vi "Load_Firmware.vi"(3 "Task":enum16{"Get Version", "Replace"}(ring), 5 "Bot Settings":T1) -> (0 "error out":errorcluster, 1 "Version":dbl, 2 "standard error":string)   [LabVIEW 2012]
uses:
  <userlib>/BotSpeak/VIs/Direct/BotSpeak_Control.ctl
panel:
  out "password":string
  out "return code":i32
  out "address":string="192.168.7.2"
  out "username":string="root"
  out "filenames":string[](array[string])=["BotSpeak2.js", "BotSpeak3.js", "BotSpeak4.js"]
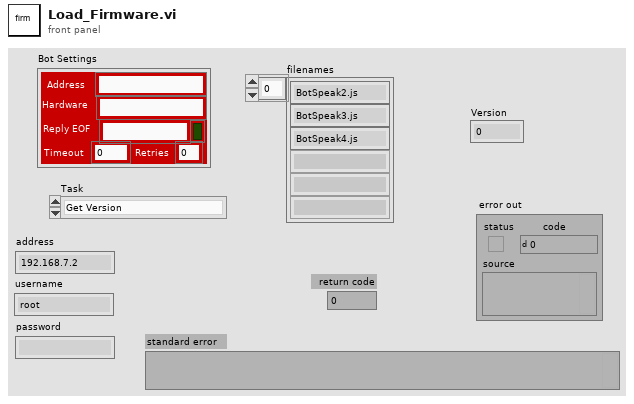
[diagram p1: front panel]
types:
  T1 = typedef "BotSpeak_Control.ctl" = cluster{"Address":string, "Reply EOF":string, "Hardware":string, "Retries":i8, "Timeout":i32, "Open?":bool}
  T2 = typedef "BotSpeak.HardwareSpecs.ctl" = cluster{"Hardware Name":string, "Hardware URL":string, "ComType":enum16{"Undefined", "Serial", "TCPIP", "Console", "EV3"}, "TCP Port":i32, "DefaultAddress":string, "Retries":i32, "Translate":enum16{"None", "Tiny", "URAPI"}, "MaxScriptSize":i32, "MaxVarNumber":i32, "StartupWait":i32, "Patience":i32, "Startup Patience":i32, "Hardware Help":string, "Com Protocol":string, "Translator":cluster{"BotSpeak CMD":string, "CMD out":string}[], "Init Code":string, "Variable Format":enum16{"INT", "FLOAT", "FIXED"}, "username":string, "password":string}
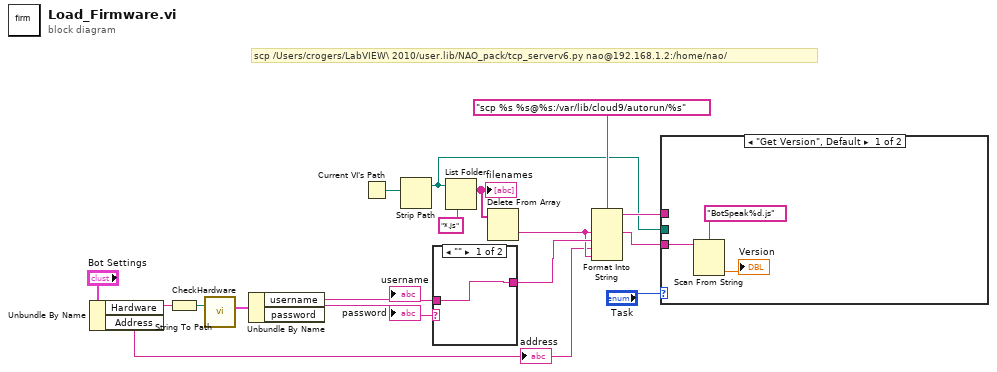
[diagram p0: block diagram]
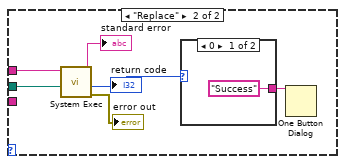
[diagram p2: hidden frame]
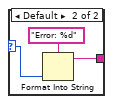
[diagram p3: hidden frame]
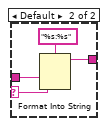
[diagram p4: hidden frame]
diagram:
  # "scp /Users/crogers/LabVIEW\\ 2010/user.lib/NAO_pack/tcp_serverv6.py nao@192.168.1.2:/home/nao/"
  n1 = Unbundle By Name("Bot Settings") -> ("Hardware"=w7:string, "Address"=w1:string)
  "address" <- w1
  n2 = String To Path(string=w7) -> (path=w6:path)
  n3 = call <userlib>:"CheckHardware.vi"("Hardware"=w6) -> ("HardwareSpecs"=w4:T2)  [unwired: 2 in]
  n4 = Unbundle By Name(w4) -> ("username"=w3:string, "password"=w2:string)
  "username" <- w3
  "password" <- w2
  n5 = Current VI's Path() -> (path=w16:path)
  n6 = Strip Path(path=w16) -> (stripped path=w11:path)  [unwired: 1 out]
  n7 = case shown="\"\"" w2 {
    selector: w2 -> [_ w20]
    tunnel: w3 -> [w17 w19]
    tunnel: [w17 w18] -> w10
    frame "" {
    }
    frame Default {
      n8 = Format Into String(format string="%s:%s", w19, w20) -> (resulting string=w18:string)  [unwired: 2 in, 1 out]
    }
  }
  n9 = List Folder(path=w11, pattern="*.js") -> (filenames=w14:string[])  [unwired: 2 in, 3 out]
  "filenames" <- w14
  n10 = Delete From Array(array=w14) -> (deleted portion=w8:string)  [unwired: 2 in, 1 out]
  n11 = Format Into String(format string="scp %s %s@%s:/var/lib/cloud9/autorun/%s", w8, w10, w1, w8) -> (resulting string=w12:string)  [unwired: 2 in, 1 out]
  n12 = case shown="\"Get Version\", Default" "Task" {
    tunnel: w12 -> [_ w30]
    tunnel: w11 -> [_ w29]
    tunnel: w8 -> [w24 _]
    frame "Get Version", Default {
      n13 = Scan From String(format string="BotSpeak%d.js", input string=w24) -> (output 1=→"Version":dbl)  [unwired: 3 in, 3 out]
    }
    frame "Replace" {
      n14 = call <vilib>:"System Exec.vi"("working directory"=w29, "command line"=w30) -> ("error out"=→"error out":errorcluster, "return code"=w26:i32, "standard error"=→"standard error":string)  [unwired: 6 in, 1 out]
      "return code" <- w26
      n15 = case shown="0" w26 {
        selector: w26 -> [_ w33]
        tunnel: ["Success" w32] -> w25
        frame 0 {
        }
        frame Default {
          n16 = Format Into String(format string="Error: %d" ("message"), w33) -> (resulting string=w32:string)  [unwired: 2 in, 1 out]
        }
      }
      n17 = One Button Dialog(message=w25) -> ()  [unwired: 1 in, 1 out]
    }
  }
